vi "zmq_curve_pair.vi"(8 "error in":errorcluster, 11 "secret in":string) -> (0 "error out":errorcluster, 2 "public out":string, 3 "secret out":string)   [LabVIEW 2025, in "ZeroMQ.lvlib"]
doc: "Generates a key pair for curve encryption. If a secret key is provided, the corresponding public key is generated. Otherwise a new pair of secret and public keys will be constructed.\n\nDetailed API documentation: http://api.zeromq.org/master:zmq-curve-keypair"
uses:
  ZeroMQ.lvlib
  libzmq-v143-mt-4_3_6/LibZMQ.lvlib
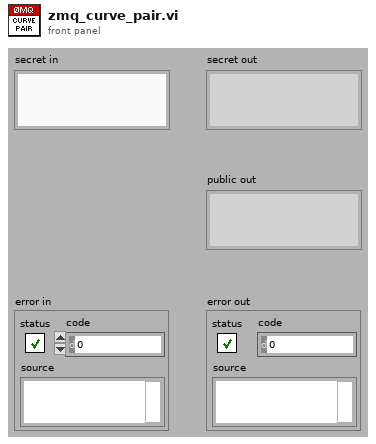
[diagram p1: front panel]
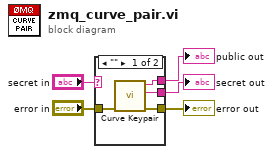
[diagram p0: block diagram]
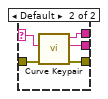
[diagram p2: hidden frame]
diagram:
  n1 = case shown="\"\"" "secret in" {
    selector: "secret in" -> [_ w14]
    tunnel: [w9 w12] -> w2
    tunnel: [w8 w13] -> w1
    tunnel: [w7 w10] -> w4
    tunnel: "error in" -> [w6 w11]
    frame "" {
      n2 = call "Curve Keypair.vi"("error in (no error)"=w6) -> ("error out"=w7:errorcluster, "z85_secret_key_ out"=w8:string, "z85_public_key_ out"=w9:string)  [unwired: 8 in]
    }
    frame Default {
      n3 = call "Curve Keypair.vi"("error in (no error)"=w11, "z85_secret_key_"=w14) -> ("error out"=w10:errorcluster, "z85_secret_key_ out"=w13:string, "z85_public_key_ out"=w12:string)  [unwired: 7 in]
    }
  }
  "error out" <- w4
  "public out" <- w2
  "secret out" <- w1
